vi "SetControlRef.vi"(8 "error in (no error)":errorcluster, 10 "Ctl Ref":refnum<vi>, 11 "reference in":refnum<class "TestView_Tree_Single.lvclass">) -> (0 "error out":errorcluster, 3 "reference in":refnum<class "TestView_Tree_Single.lvclass">)   [LabVIEW 2022 SP3, in "TestView_Tree_Single.lvlib" / "TestView_Tree_Single.lvclass"]
uses:
  TestView_Tree_Single.lvclass
  TestType.ctl
  Components/ViPER.lvlibp/ViPER.lvclass
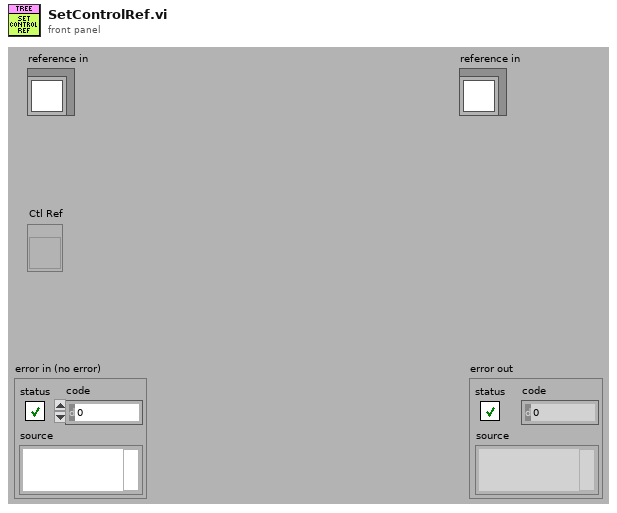
[diagram p1: front panel]
types:
  T1 = enum32{"None", "LabVIEW", "Mac OS", "Windows", "Default"}
  T2 = typedef "TestView_Tree_Single.lvlib/TestView_Tree_Single.lvclass/TestType.ctl" = enum16{"null", "action", "action_active", "action_done", "group", "group_active", "group_fail", "group_pass", "test", "test_active", "test_fail", "test_pass", "warning"}
  T3 = typedef "TestView_Tree_Single.lvlib/TestView_Tree_Single.lvclass/ObjectAttributes.ctl" = cluster{"Front Panel":refnum<vi>, "Last_Item":string, "Config":T4, "Title":string, "User":string, "TreeRef":refnum<vi>, "Active DUT":i32, "Status":T5, "SN":string, "Spec":string}
  T4 = typedef "TestView_Tree_Single.lvlib/TestView_Tree_Single.lvclass/Config.ctl" = cluster{"default":string}
  T5 = typedef "TestView_Base.lvlibp/TestView_Base.lvclass/ViewStatus.ctl" = enum16{"Testing", "Ready", "Logout", "Login", "PASS", "FAIL", "FAULT", "ABORTED"}
  T6 = typedef "imagedata.ctl" = cluster{"image type":i32, "image depth":i32, "image":u8[], "mask":u8[], "colors":u32[], "Rectangle":cluster{"left":i16, "top":i16, "right":i16, "bottom":i16}}
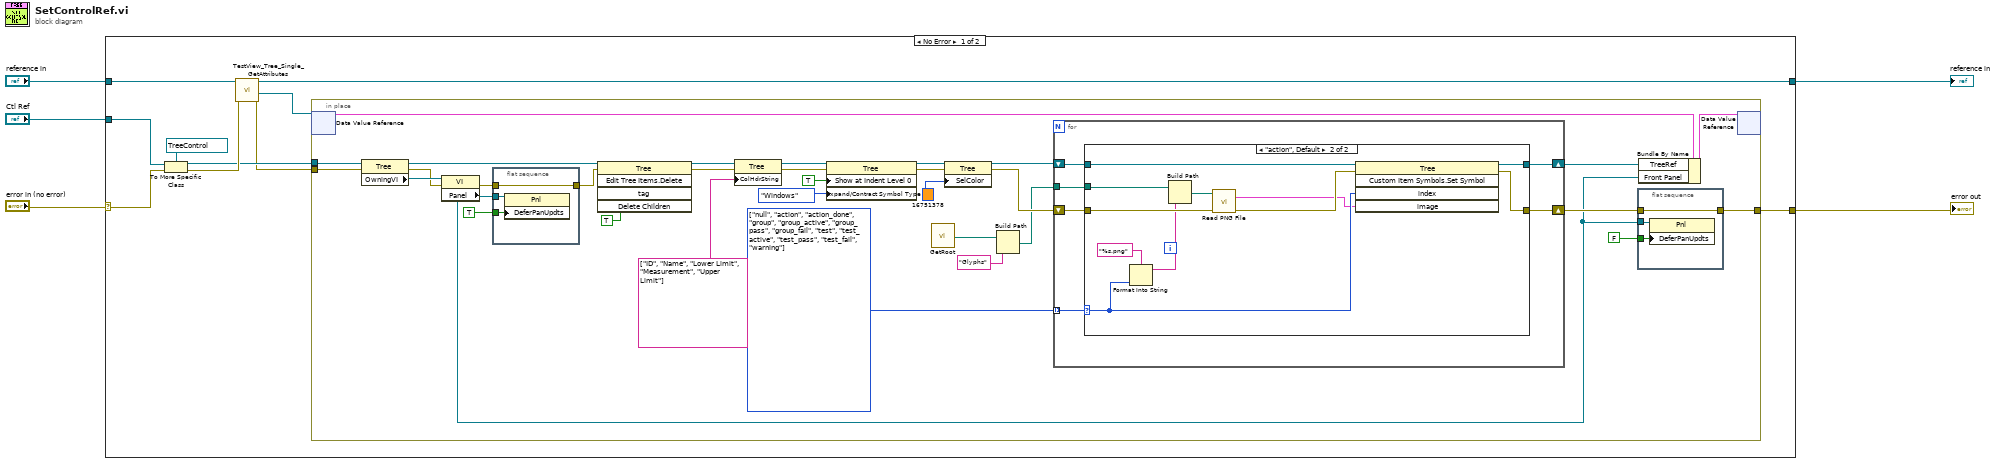
[diagram p0: block diagram]
diagram:
  n1 = case shown="No Error" "error in (no error)" {
    selector: "error in (no error)" -> [w8 w74]
    tunnel: [w6 w74] -> w4
    tunnel: [w7 w73] -> w2
    tunnel: "reference in" -> [w9 w73]
    tunnel: "Ctl Ref" -> [w14 _]
    frame No Error {
      n2 = To More Specific Class(target class=refnum<vi> refnum ("Tree ref"), reference=w14, error in=w8) -> (specific class reference=w12:refnum<vi>, error out=w13:errorcluster)
      n3 = call "TestView_Tree_Single_GetAttributes.vi"("error in (no error)"=w13, "reference in"=w9) -> ("error out"=w10:errorcluster, "DataRef"=w11:refnum<data-value>, "reference out"=w7:refnum<class "TestView_Tree_Single.lvclass">)  [unwired: 6 in, 1 out]
      n4 = in-place {
        in-place-border: w10 -> [w29]
        in-place-border: [w23] -> w6
        in-place-border: w12 -> [w18]
        w35 = T2[] [enum."null", enum."action", enum."action_done", enum."group", enum."group_active", enum."group_pass", enum."group_fail", enum."test", enum."test_active", enum."test_pass", enum."test_fail", enum."warning"] items=["null", "action", "action_active", "action_done", "group", "group_active", "group_fail", "group_pass", "test", "test_active", "test_fail", "test_pass", "warning"]
        n5 = in-place-dvr #1(w11) -> (w21:T3)  [unwired: 1 out]
        n6 = property class="Tree"(reference=w18, error in=w29) -> (reference out=w32:refnum<vi>, error out=w30:errorcluster, "OwningVI"=w31:refnum<vi>)
        n7 = property class="VI"(reference=w31, error in=w30) -> (error out=w27:errorcluster, "Panel"=w22:refnum<vi>)  [unwired: 1 out]
        n8 = flat-sequence {
          tunnel: w22 -> [w53]
          tunnel: TRUE ("Defer Panel Updates") -> [w52]
          tunnel: w27 -> [w51]
          tunnel: [w51] -> w26
          frame #0 {
            n9 = property class="Pnl"(reference=w53, "DeferPanUpdts"=w52) -> ()  [unwired: 1 in, 2 out]
          }
        }
        n10 = invoke class="Tree" method="Edit Tree Items.Delete"(reference=w32, error in=w26, "Delete Children"=TRUE ("Delete Children?")) -> (reference out=w45:refnum<vi>, error out=w44:errorcluster)  [unwired: 2 in, 3 out]
        n11 = property class="Tree"(reference=w45, error in=w44, "ColHdrString"=string[] ["ID", "Name", "Lower Limit", "Measurement", "Upper Limit"] ("Column Header Strings[]")) -> (reference out=w41:refnum<vi>, error out=w40:errorcluster)
        n12 = property class="Tree"(reference=w41, error in=w40, "Show at Indent Level 0"=TRUE ("Expand/Contract Symbol:Show Symbol at Root"), "Expand/Contract Symbol Type"=T1."Windows" ("Expand/Contract Symbol:Symbol Type")) -> (reference out=w38:refnum<vi>, error out=w36:errorcluster)
        n13 = call "GetRoot.vi"() -> ("Root"=w16:path)  [unwired: 10 in, 1 out]
        n14 = property class="Tree"(reference=w38, error in=w36, "SelColor"=u32 16751378 ("Color Box")) -> (reference out=w33:refnum<vi>, error out=w34:errorcluster)
        n15 = Build Path(base path=w16, name or relative path="Glyphs") -> (appended path=w19:path)
        n16 = for {
          tunnel: w19 -> [w59]
          tunnel: w35 -> [w54] mode=indexing
          shift-right: [w55] -> w17
          shift-left: w33 -> [w57]
          shift-right: [w56] -> w24
          shift-left: w34 -> [w58]
          n17 = case shown="\"action\", Default" w54 {
            selector: w54 -> [_ w65]
            tunnel: w59 -> [_ w72]
            tunnel: w58 -> [w60 w70]
            tunnel: w57 -> [w61 w69]
            tunnel: [w60 w67] -> w56
            tunnel: [w61 w66] -> w55
            frame "null" {
            }
            frame "action", Default {
              n18 = Format Into String(format string="%s.png", w65) -> (resulting string=w63:string)  [unwired: 2 in, 1 out]
              n19 = Build Path(base path=w72, name or relative path=w63) -> (appended path=w71:path)
              n20 = call <vilib>:"Read PNG File.vi"("error in (no error)"=w70, "path to PNG file"=w71) -> ("error out"=w68:errorcluster, "image data"=w62:T6)  [unwired: 7 in, 1 out]
              n21 = invoke class="Tree" method="Custom Item Symbols.Set Symbol"(reference=w69, error in=w68, "index"=w65, "image"=w62) -> (reference out=w66:refnum<vi>, error out=w67:errorcluster)  [unwired: 1 in, 3 out]
            }
          }
        }
        n22 = flat-sequence {
          tunnel: w22 -> [w50]
          tunnel: FALSE ("Defer Panel Updates") -> [w49]
          tunnel: w24 -> [w48]
          tunnel: [w48] -> w23
          frame #0 {
            n23 = property class="Pnl"(reference=w50, "DeferPanUpdts"=w49) -> ()  [unwired: 1 in, 2 out]
          }
        }
        n24 = Bundle By Name(cluster=w21, "TreeRef"=w17, "Front Panel"=w22) -> (w47:T3)
        n25 = in-place-dvr #1(w47) -> ()  [unwired: 2 out]
      }
    }
    frame Error {
    }
  }
  "error out" <- w4
  "reference in" <- w2
